vi "Get File Extension.vi"(11 "Filename":string) -> (2 "Lowercase Extension":string, 3 "Filename without Extension":string)   [LabVIEW 2020, in "VI Properties Editor.lvlib" / "Project Tree Map.lvclass"]
doc: "Gets the file extension of <B>Filename</B>, without the leading period."
uses:
  Project Tree Map.lvclass
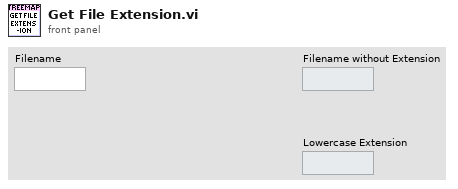
[diagram p1: front panel]
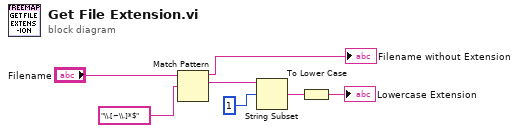
[diagram p0: block diagram]
diagram:
  n1 = Match Pattern(string="Filename", regular expression="\\.[~\\.]*$") -> (before substring=→"Filename without Extension":string, match substring=w5:string)  [unwired: 3 out]
  n2 = String Subset(string=w5, offset (0)=1) -> (substring=w4:string)  [unwired: 1 out]
  n3 = To Lower Case(string=w4) -> (all lower case string=→"Lowercase Extension":string)
